vi "Main.vi"(11 "Module Admin":refnum<class "Delacor_lib_QMH_Module Admin.lvclass">) -> ()   [LabVIEW 2018, in "DAQ.lvlib"]
doc: "This template is based off of the Queued Message Handler design pattern and the Queued Message Handler project template that ships with LabVIEW.\n\nThe main difference is that the queue is private to this module and communication between modules is performed via Broadcast and Request events.\n\nRequest events are wrapped in public API methods and are handled in the Event Handling Loop (EHL) of this VI. Any module can register for Broadcast events sent by this module. The EHL generates messages based on user interface actions.\n\nThe Message Handling Loop (MHL) processes messages generated by the EHL, or by other messages. The messages are string values, so new messages can be added easily to the Message Cases case structure in the MHL. Each message cluster can also provide an optional value for Message Data, which is a variant that can be converted to whatever message-specific data is required.\n_____\nBased on DQMH Project Template 6.1.0.94."
uses:
  DAQ.lvlib
  <vilib>/Delacor/Delacor QMH/Libraries/Module Admin_class/Delacor_lib_QMH_Module Admin.lvclass
  Module Data--cluster.ctl
  <vilib>/Modbus/master/Modbus Master.lvclass
  <vilib>/Delacor/Delacor QMH/Libraries/Message Queue_class/Delacor_lib_QMH_Message Queue.lvclass/Delacor_lib_QMH_Message Queue.ctl
  Stop Argument--cluster.ctl
  <vilib>/Delacor/Delacor QMH/Libraries/Module Admin_class/Delacor_lib_QMH_Module Admin.lvclass/Delacor_lib_QMH_Module Admin.ctl
  Update Sampling Rate Argument--cluster.ctl
  <vilib>/Utility/miscctls.llb/LVPointTypeDef.ctl
  <vilib>/Delacor/Delacor QMH/Libraries/Message Queue_class/Delacor_lib_QMH_Enqueue Message (Single).vi
  <vilib>/Delacor/Delacor QMH/Libraries/Module Admin_class/Delacor_lib_QMH_Get External Launch.vi
  <vilib>/Delacor/Delacor QMH/Libraries/Message Queue_class/Delacor_lib_QMH_Enqueue Message (Array).vi
  <vilib>/Utility/error.llb/Error Cluster From Error Code.vi
  <vilib>/ErrorRing/Error Ring.xnode
  <vilib>/Delacor/Delacor QMH/Libraries/Message Queue_class/Delacor_lib_QMH_Message Queue.lvclass
panel:
  out "Message":string
  out "error out":errorcluster
  out "Status":string
  in  "Simulate MHL Error":bool
  in  "Simulate EHL Error":bool
  # "Other QMH Modules communicate with this Module via its Public API (wrappers for its Request Events).\n\nThis Module communicates with other Modules via its Broadcast Events.\nAny module that wants to get these messages, just registers for this module's Broadcast events."
  # "This template is for the Delacor Modified Queued Message Handler design pattern.\n\nSee the block diagram for more information on how to use this template."
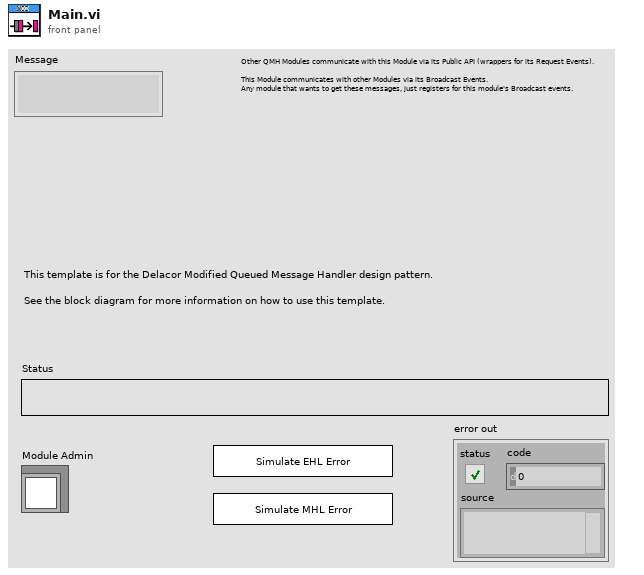
[diagram p1: front panel]
types:
  T1 = typedef "DAQ.lvlib/Request Events--cluster.ctl" = cluster{"Stop Module":refnum<user-event>, "Show Panel":refnum<user-event>, "Hide Panel":refnum<user-event>, "Get Module Execution Status":refnum<user-event>, "Show Diagram":refnum<user-event>, "Wakeup or Sleep HL":refnum<user-event>, "建立连接":refnum<user-event>, "断开连接":refnum<user-event>, "Update Sampling Rate":refnum<user-event>}
  T2 = typedef "DAQ.lvlib/Module Data--cluster.ctl" = cluster{"Status":string, "Mod":cluster{"Con?":bool, "主设备":refnum<class "Modbus Master.lvclass">}, "Sampling Rate":i32}
  T3 = enum32{"invalid lock state", "Not Locked", "Locked (No Password)", "Password-protected"}
  T4 = typedef "DAQ.lvlib/Stop Argument--cluster.ctl" = cluster{"Origin":string, "Exit via Stop Module Req?":bool, "Wait for Module to stop?":bool}
  T5 = typedef "DAQ.lvlib/建立连接 Argument--cluster.ctl" = cluster{"Mod ID":i32}
  T6 = typedef "DAQ.lvlib/断开连接 Argument--cluster.ctl" = cluster{"Mod ID":i32}
  T7 = typedef "DAQ.lvlib/Update Sampling Rate Argument--cluster.ctl" = cluster{"Sampling Rate":i32}
  T8 = typedef "LVPointTypeDef.ctl" = cluster{"Horizontal":i16, "Vertical":i16}
  T9 = enum32{"Invalid", "Standard", "Closed", "Hidden", "Minimized", "Maximized"}
  T10 = cluster{"Con?":bool, "主设备":refnum<class "Modbus Master.lvclass">}
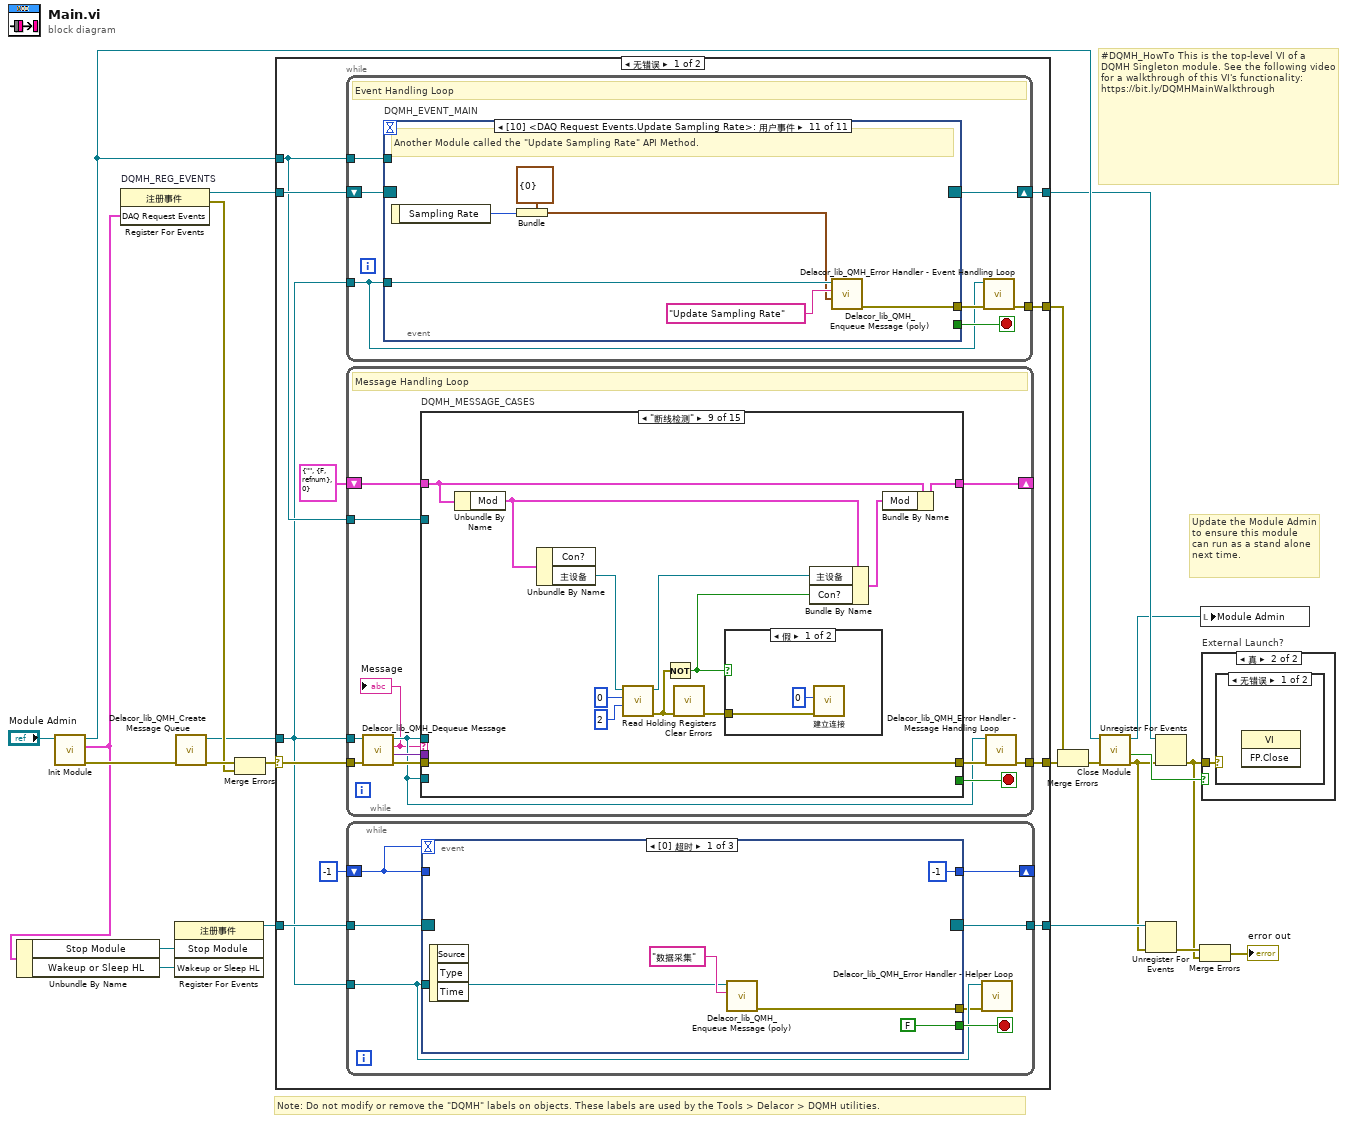
[diagram p0: block diagram]
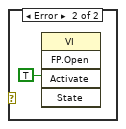
[diagram p3: hidden frame]
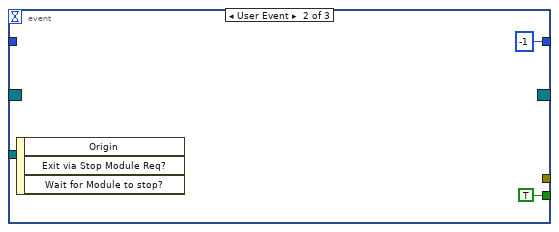
[diagram p4: hidden frame]
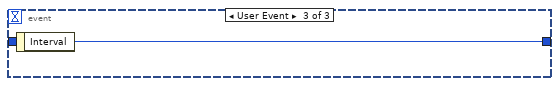
[diagram p5: hidden frame]
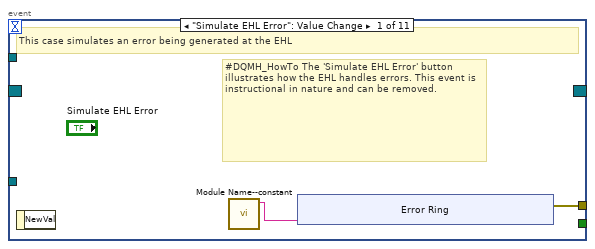
[diagram p6: hidden frame]
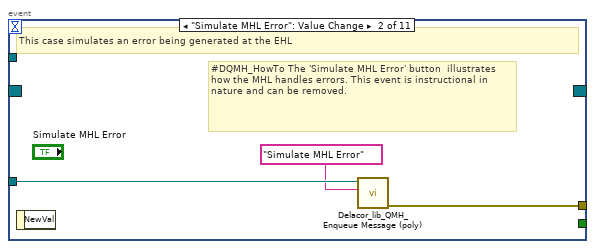
[diagram p7: hidden frame]
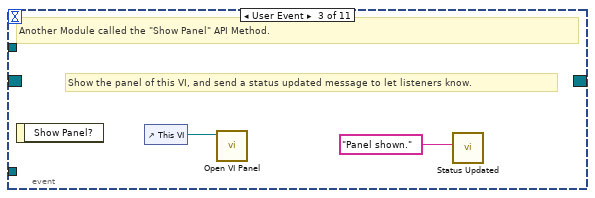
[diagram p8: hidden frame]
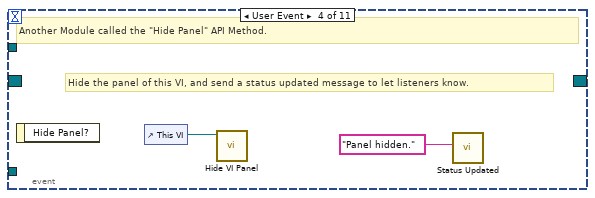
[diagram p9: hidden frame]
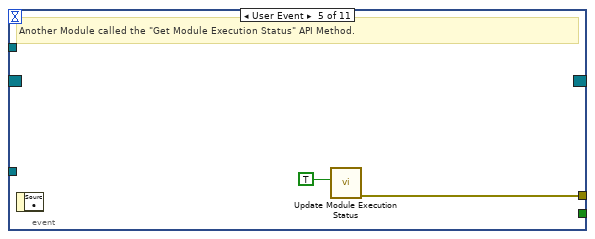
[diagram p10: hidden frame]
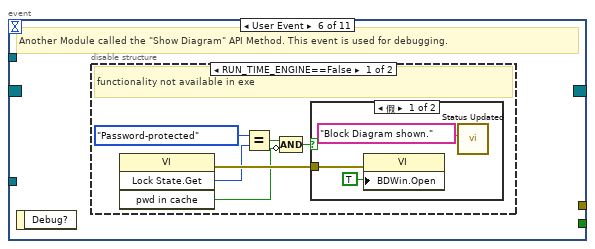
[diagram p11: hidden frame]
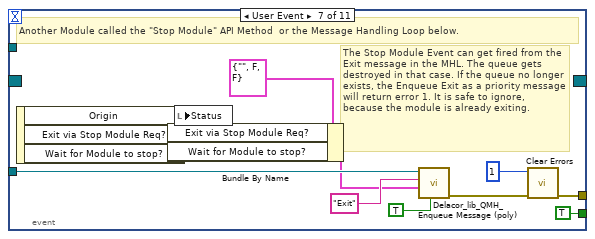
[diagram p14: hidden frame]
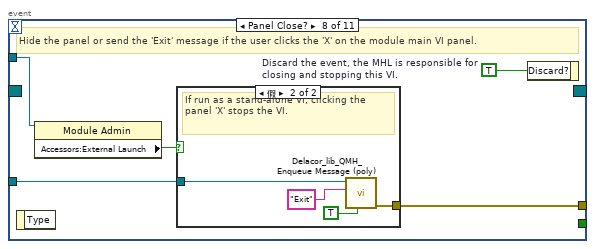
[diagram p15: hidden frame]
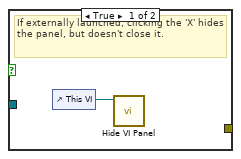
[diagram p16: hidden frame]
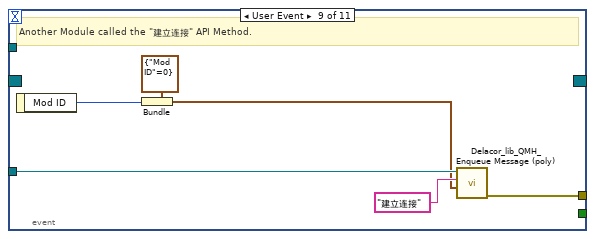
[diagram p17: hidden frame]
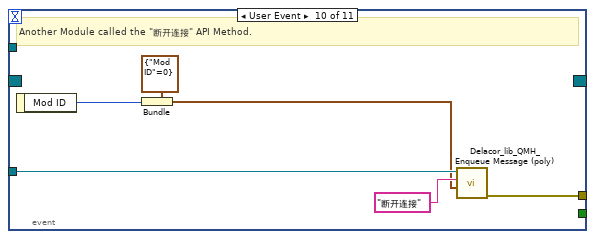
[diagram p18: hidden frame]
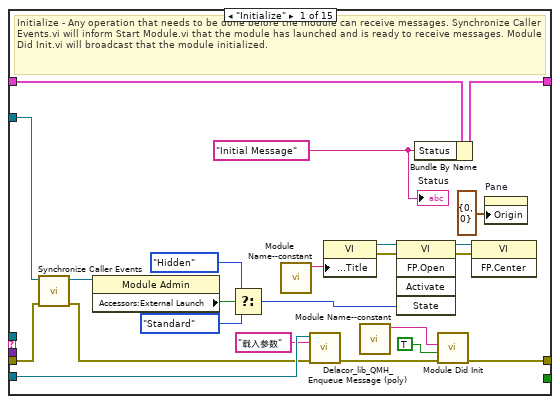
[diagram p19: hidden frame]
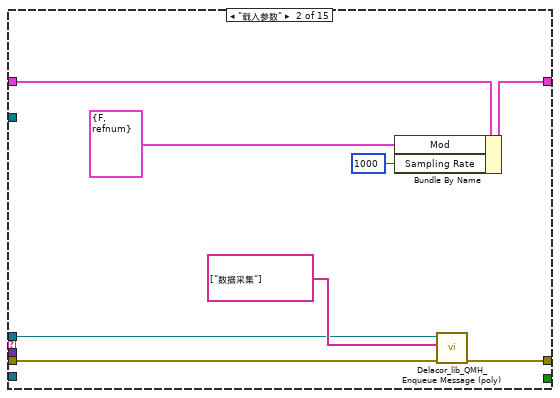
[diagram p20: hidden frame]
diagram:
  # "#DQMH_HowTo This is the top-level VI of a DQMH Singleton module. See the following video for a walkthrough of this VI's functionality: https://bit.ly/DQMHMainWalkthrough"
  # "Note: Do not modify or remove the \"DQMH\" labels on objects. These labels are used by the Tools > Delacor > DQMH utilities."
  # "Update the Module Admin to ensure this module can run as a stand alone next time."
  n1 = call "Init Module.vi"("Singleton Module Admin in"="Module Admin") -> ("error out"=w22:errorcluster, "DAQ Request Events"=w5:T1, "Singleton Module Admin out"=w16:refnum<class "Delacor_lib_QMH_Module Admin.lvclass">)  [unwired: 8 in]
  n2 = Unbundle By Name ("按名称解除捆绑")(w5) -> ("Stop Module"=w8:refnum<user-event>, "Wakeup or Sleep HL"=w7:refnum<user-event>)
  n3 = register-events "DQMH_REG_EVENTS"(w5) -> (reference out=w14:refnum<event-registration>, error out=w17:errorcluster)  [unwired: 2 in]
  n4 = register-events ("注册事件")(w8, w7) -> (reference out=w6:refnum<event-registration>)  [unwired: 2 in, 1 out]
  n5 = call <vilib>:"Delacor_lib_QMH_Create Message Queue.vi"("error in"=w22) -> ("error out"=w19:errorcluster, "Message Queue"=w13:refnum<class "Delacor_lib_QMH_Message Queue.lvclass">)  [unwired: 9 in]
  n6 = Merge Errors(w19, w17) -> (w18:errorcluster)
  n7 = case shown="无错误" w18 {
    selector: w18 -> [w32 w296]
    tunnel: [w34 w295] -> w23
    tunnel: [w31 w301] -> w15
    tunnel: w14 -> [w29 w301]
    tunnel: w13 -> [w25 w294]
    tunnel: [w33 _] -> w21
    tunnel: w16 -> [w28 w297]
    tunnel: w6 -> [w26 w293]
    tunnel: [w24 w293] -> w4
    frame No Error {
      n8 = while {
        tunnel: w25 -> [w50]
        shift-right: [w53] -> w31
        shift-left: w29 -> [w54]
        tunnel: [w55] -> w33
        tunnel: w28 -> [w51]
        stop <- w52 stop-if-true
        # "Event Handling Loop"
        n9 = event "DQMH_EVENT_MAIN" shown="[10] <DAQ Request Events.Update Sampling Rate>: 用户事件" {
          selector: w54 -> [_ _ _ _ _ _ _ _ _ _ _]
          dyn-events: [_ _ _ _ _ _ _ _ _ _ _] -> w53
          timeout: _ -> [_ _ _ _ _ _ _ _ _ _ _]
          tunnel: [_ _ _ _ _ _ TRUE ("Discard?") _ _ _ _] -> w52
          tunnel: w50 -> [_ w67 _ _ _ _ w91 w98 w111 w117 w123]
          tunnel: [w58 w68 _ _ w74 _ w94 w100 w106 w112 w118] -> w56
          tunnel: w51 -> [_ _ _ _ _ _ _ w97 _ _ _]
          event "Simulate EHL Error": Value Change {
            # "#DQMH_HowTo The 'Simulate EHL Error' button  illustrates how the EHL handles errors. This event is instructional in nature and can be removed."
            # "This case simulates an error being generated at the EHL"
            n10 = event-data() -> ()  [unwired: 1 in, 1 out]
            n11 = call "Module Name--constant.vi"() -> ("Module Name"=w57:string)  [unwired: 11 in]
            n12 = xnode "Error Ring"("参数 0"=w57) -> ("错误输出"=w58:errorcluster)
          }
          event "Simulate MHL Error": Value Change {
            # "#DQMH_HowTo The 'Simulate MHL Error' button  illustrates how the MHL handles errors. This event is instructional in nature and can be removed."
            # "This case simulates an error being generated at the EHL"
            n13 = event-data() -> ()  [unwired: 1 in, 1 out]
            n14 = call-poly <vilib>:"Delacor_lib_QMH_Enqueue Message (poly).vi"("Message"="Simulate MHL Error", "Message Queue in"=w67) -> ("error out"=w68:errorcluster)  [unwired: 8 in, 1 out]
          }
          event User Event {
            # "Show the panel of this VI, and send a status updated message to let listeners know."
            # "Another Module called the \"Show Panel\" API Method."
            n15 = event-data() -> ()  [unwired: 1 in, 1 out]
            n16 = control-ref of="This VI"() -> (w70:refnum<vi>)
            n17 = call "Open VI Panel.vi"("VI"=w70) -> ()  [unwired: 10 in, 1 out]
            n18 = call "Status Updated.vi"("Status"="Panel shown." ("format string")) -> ()  [unwired: 10 in, 1 out]
          }
          event User Event {
            # "Hide the panel of this VI, and send a status updated message to let listeners know."
            # "Another Module called the \"Hide Panel\" API Method."
            n19 = event-data() -> ()  [unwired: 1 in, 1 out]
            n20 = control-ref of="This VI"() -> (w72:refnum<vi>)
            n21 = call "Hide VI Panel.vi"("VI"=w72) -> ()  [unwired: 10 in, 1 out]
            n22 = call "Status Updated.vi"("Status"="Panel hidden." ("format string")) -> ()  [unwired: 10 in, 1 out]
          }
          event User Event {
            # "Another Module called the \"Get Module Execution Status\" API Method."
            n23 = event-data() -> ()  [unwired: 1 in, 1 out]
            n24 = call "Update Module Execution Status.vi"("Running?"=TRUE) -> ("error out"=w74:errorcluster)  [unwired: 10 in]
          }
          event User Event {
            # "Another Module called the \"Show Diagram\" API Method. This event is used for debugging."
            n25 = event-data() -> ()  [unwired: 1 in, 1 out]
            n26 = disable-structure shown="RUN_TIME_ENGINE==False" {
              frame condition #0 (active) {
                # "functionality not available in exe"
                n27 = invoke class="VI" method="Lock State.Get"() -> (error out=w80:errorcluster, "Get Lock State"=w79:T3, "pwd in cache"=w76:bool)  [unwired: 4 in, 1 out]
                n28 = Equal?(x=T3."Password-protected", y=w79) -> (x = y?=w77:bool)
                n29 = Compound Arithmetic op=AND(w77, invert w76) -> (w75:bool)
                n30 = case "条件结构" shown="假" w75 {
                  tunnel: w80 -> [w83 _]
                  frame False {
                    n31 = property class="VI"(error in=w83, "BDWin.Open"=TRUE ("Block Diagram Window:Open")) -> ()  [unwired: 1 in, 2 out]
                    n32 = call "Status Updated.vi"("Status"="Block Diagram shown." ("format string")) -> ()  [unwired: 10 in, 1 out]
                  }
                  frame True {
                    # "Password-protected VI, and the password is not in the cache. Do not show the diagram."
                  }
                }
              }
              frame condition #1 {
              }
            }
          }
          event User Event {
            # "The Stop Module Event can get fired from the Exit message in the MHL. The queue gets destroyed in that case. If the queue no longer exists, the Enqueue Exit as a priority message will return error 1. It is safe to ignore, because the module is already exiting."
            # "Another Module called the \"Stop Module\" API Method  or the Message Handling Loop below."
            n33 = event-data() -> ("Origin"=w90:string, "Exit via Stop Module Req?"=w86:bool, "Wait for Module to stop?"=w85:bool)  [unwired: 1 in]
            n34 = Bundle By Name(cluster=T4 {"Origin"="", "Exit via Stop Module Req?"=FALSE, "Wait for Module to stop?"=FALSE} ("Stop Argument"), "Exit via Stop Module Req?"=w86, "Wait for Module to stop?"=w85) -> (w84:T4)
            n35 = local write "Status"(w90) -> ()
            n36 = call-poly <vilib>:"Delacor_lib_QMH_Enqueue Message (poly).vi"("Priority Message? (F)"=TRUE, "Message Data"=w84, "Message"="Exit", "Message Queue in"=w91) -> ("error out"=w95:errorcluster)  [unwired: 6 in, 1 out]
            n37 = call <vilib>:"Clear Errors.vi"("error in (no error)"=w95, "specific error code to clear (0: all)"=1) -> ("error out"=w94:errorcluster)  [unwired: 4 in, 1 out]
          }
          event Panel Close? {
            w99 = TRUE  # Discard the event, the MHL is responsible for closing and stopping this VI.
            # "Hide the panel or send the 'Exit' message if the user clicks the 'X' on the module main VI panel."
            n38 = event-data() -> ()  [unwired: 1 in, 1 out]
            n39 = property class="Module Admin"(reference=w97) -> ("Accessors:External Launch"=w96:bool)  [unwired: 1 in, 2 out]
            n40 = case "条件结构" shown="假" w96 {
              tunnel: w98 -> [_ w104]
              tunnel: [_ w105] -> w100
              frame True {
                # "If externally launched, clicking the 'X' hides the panel, but doesn't close it."
                n41 = control-ref of="This VI"() -> (w101:refnum<vi>)
                n42 = call "Hide VI Panel.vi"("VI"=w101) -> ()  [unwired: 10 in, 1 out]
              }
              frame False {
                # "If run as a stand-alone VI, clicking the panel 'X' stops the VI."
                n43 = call-poly <vilib>:"Delacor_lib_QMH_Enqueue Message (poly).vi"("Priority Message? (F)"=TRUE, "Message"="Exit", "Message Queue in"=w104) -> ("error out"=w105:errorcluster)  [unwired: 7 in, 1 out]
              }
            }
            n44 = event-data("Discard?"=w99) -> ()  [unwired: 1 in, 1 out]
          }
          event User Event {
            # "Another Module called the \"建立连接\" API Method."
            n45 = event-data() -> ("Mod ID"=w107:i32)  [unwired: 1 in]
            n46 = Bundle(cluster=T5 {"Mod ID"=0} ("建立连接 Argument"), "Mod ID"=w107) -> (w108:T5)
            n47 = call-poly <vilib>:"Delacor_lib_QMH_Enqueue Message (poly).vi"("Message Data"=w108, "Message"="建立连接", "Message Queue in"=w111) -> ("error out"=w106:errorcluster)  [unwired: 7 in, 1 out]
          }
          event User Event {
            # "Another Module called the \"断开连接\" API Method."
            n48 = event-data() -> ("Mod ID"=w113:i32)  [unwired: 1 in]
            n49 = Bundle(cluster=T6 {"Mod ID"=0} ("断开连接 Argument"), "Mod ID"=w113) -> (w114:T6)
            n50 = call-poly <vilib>:"Delacor_lib_QMH_Enqueue Message (poly).vi"("Message Data"=w114, "Message"="断开连接", "Message Queue in"=w117) -> ("error out"=w112:errorcluster)  [unwired: 7 in, 1 out]
          }
          event User Event {
            # "Another Module called the \"Update Sampling Rate\" API Method."
            n51 = event-data() -> ("Sampling Rate"=w119:i32)  [unwired: 1 in]
            n52 = Bundle(cluster=T7 {"Sampling Rate"=0} ("Update Sampling Rate Argument"), "Sampling Rate"=w119) -> (w120:T7)
            n53 = call-poly <vilib>:"Delacor_lib_QMH_Enqueue Message (poly).vi"("Message Data"=w120, "Message"="Update Sampling Rate", "Message Queue in"=w123) -> ("error out"=w118:errorcluster)  [unwired: 7 in, 1 out]
          }
        }
        n54 = call-dynamic "Delacor_lib_QMH_Error Handler - Event Handling Loop.vi"("error in"=w56, "Message Queue in"=w50) -> ("dup error in"=w55:errorcluster)  [unwired: 8 in, 1 out]
      }
      n55 = while {
        tunnel: w25 -> [w127]
        shift-right: [w130] -> _
        shift-left: T2 {"Status"="", "Mod"={"Con?"=FALSE, "主设备"=refnum}, "Sampling Rate"=0} ("Data Cluster") -> [w131]
        tunnel: w32 -> [w134]
        tunnel: [w132] -> w34
        tunnel: w28 -> [w126]
        stop <- w129 stop-if-true
        # "Message Handling Loop"
        n56 = call-dynamic "Delacor_lib_QMH_Dequeue Message.vi"("error in"=w134, "Message Queue in"=w127) -> ("error out"=w133:errorcluster, "Message Data"=w128:variant, "Message"=w124:string, "Message Queue out"=w125:refnum<class "Delacor_lib_QMH_Message Queue.lvclass">)  [unwired: 6 in]
        "Message" <- w124
        n57 = case "DQMH_MESSAGE_CASES" shown="\"断线检测\"" w124 {
          selector: w124 -> [_ _ _ _ _ _ _ _ _ _ _ _ _ _ w280]
          tunnel: w125 -> [_ w162 _ _ _ _ _ w207 _ _ _ _ w247 w272 _]
          tunnel: w133 -> [w156 w161 w168 w179 w192 w200 w203 w206 w222 w228 w232 w237 w254 w278 w282]
          tunnel: [w155 w160 w168 w171 w191 w198 w202 w208 w222 w227 w232 w236 w250 w275 w283] -> w135
          tunnel: w131 -> [w146 w166 w167 w175 w187 w199 w201 w210 w221 w230 w231 w234 w249 w264 w281]
          tunnel: [w145 w165 w167 w170 w186 w194 w201 w210 w216 w226 w231 w234 w249 w264 w281] -> w130
          tunnel: [_ _ _ _ _ _ _ _ _ _ _ _ _ w271 _] -> w129
          tunnel: w128 -> [_ _ _ w178 w190 w197 _ _ _ _ _ _ w248 w270 _]
          tunnel: w126 -> [w147 _ _ _ _ _ _ _ _ _ _ _ w246 w265 _]
          tunnel: w125 -> [w139 _ _ _ _ _ _ _ _ _ _ _ _ _ _]
          frame "Initialize" {
            w141 = "Initial Message" ("Initial Message")
            # "Initialize - Any operation that needs to be done before the module can receive messages. Synchronize Caller Events.vi will inform Start Module.vi that the module has launched and is ready to receive messages. Module Did Init.vi will broadcast that the module initialized."
            n58 = call "Synchronize Caller Events.vi"("error in (no error)"=w156, "Singleton Module Admin in"=w147) -> ("error out"=w137:errorcluster, "Singleton Module Admin out"=w142:refnum<class "Delacor_lib_QMH_Module Admin.lvclass">)  [unwired: 8 in]
            n59 = property class="Module Admin"(reference=w142) -> ("Accessors:External Launch"=w151:bool)  [unwired: 1 in, 2 out]
            n60 = Select(t=T9."Hidden" ("State"), s=w151, f=T9."Standard" ("State")) -> (s? t:f=w148:T9)
            n61 = call "Module Name--constant.vi"() -> ("Module Name"=w154:string)  [unwired: 11 in]
            n62 = call-poly <vilib>:"Delacor_lib_QMH_Enqueue Message (poly).vi"("error in"=w137, "Message"="载入参数", "Message Queue in"=w139) -> ("error out"=w136:errorcluster)  [unwired: 7 in, 1 out]
            n63 = property class="VI"("Front Panel.Title"=w154) -> (reference out=w153:refnum<vi>, error out=w158:errorcluster)  [unwired: 2 in]
            n64 = call "Module Name--constant.vi"() -> ("Module Name"=w143:string)  [unwired: 11 in]
            n65 = invoke class="VI" method="FP.Open"(reference=w153, error in=w158, "State"=w148) -> (reference out=w152:refnum<vi>, error out=w157:errorcluster)  [unwired: 2 in, 3 out]
            n66 = Bundle By Name(cluster=w146, "Status"=w141) -> (w145:T2)
            n67 = call "Module Did Init.vi"("error in (no error)"=w136, "Initialized?"=TRUE, "Origin"=w143) -> ("error out"=w155:errorcluster)  [unwired: 8 in]
            n68 = invoke class="VI" method="FP.Center"(reference=w152, error in=w157) -> ()  [unwired: 1 in, 3 out]
            n69 = property on="Pane" class="Pane"("Origin"=T8 {"Horizontal"=0, "Vertical"=0}) -> ()  [unwired: 2 in, 2 out]
            "Status" <- w141
          }
          frame "载入参数" {
            n70 = Bundle By Name(cluster=w166, "Mod"=T10 {"Con?"=FALSE, "主设备"=refnum}, "Sampling Rate"=1000) -> (w165:T2)
            n71 = call-poly <vilib>:"Delacor_lib_QMH_Enqueue Message (poly).vi"("error in"=w161, "Message Array"=string[] ["数据采集"] ("Message"), "Message Queue in"=w162) -> ("error out"=w160:errorcluster)  [unwired: 7 in, 1 out]
          }
          frame "---Module Specific---" {
            # "Separator -- The following cases handle messages specific to this Module."
          }
          frame "建立连接" {
            n72 = Variant To Data(error in=w179, type=T5 {"Mod ID"=0} ("建立连接 Argument"), Variant=w178) -> (data=w176:T5, error out=w172:errorcluster)
            n73 = Unbundle By Name(w175) -> ("Mod"=w174:T10)
            n74 = Unbundle By Name(w176) -> ("Mod ID"=w173:i32)
            n75 = call "Modbus_建立连接.vi"("error in (no error)"=w172, "Mod ID"=w173, "Mod"=w174) -> ("error out"=w171:errorcluster, "Mod 2"=w169:T10)  [unwired: 7 in]
            n76 = Bundle By Name(cluster=w175, "Mod"=w169) -> (w170:T2)
          }
          frame "断开连接" {
            n77 = Variant To Data(error in=w192, type=T6 {"Mod ID"=0} ("断开连接 Argument"), Variant=w190) -> (data=w188:T6, error out=w191:errorcluster)
            n78 = Unbundle By Name(w187) -> ("Mod"=w184:T10)
            n79 = Unbundle By Name(w188) -> ()  [unwired: 1 out]
            n80 = Unbundle By Name(w184) -> ("主设备"=w185:refnum<class "Modbus Master.lvclass">)
            n81 = call-dynamic "Close.vi"("Modbus master in"=w185) -> ("error out"=w180:errorcluster)  [unwired: 10 in]
            n82 = call <vilib>:"Clear Errors.vi"("error in (no error)"=w180) -> ()  [unwired: 5 in, 2 out]
            n83 = Bundle By Name(cluster=w184, "Con?"=FALSE, "主设备"=refnum<class "Modbus Master.lvclass"> refnum ("Modbus master in")) -> (w183:T10)
            n84 = Bundle By Name(cluster=w187, "Mod"=w183) -> (w186:T2)
          }
          frame "Update Sampling Rate" {
            n85 = Variant To Data(error in=w200, type=T7 {"Sampling Rate"=0} ("Update Sampling Rate Argument"), Variant=w197) -> (data=w195:T7, error out=w198:errorcluster)
            n86 = Unbundle By Name(w195) -> ("Sampling Rate"=w193:i32)
            n87 = Bundle By Name(cluster=w199, "Sampling Rate"=w193) -> (w194:T2)
          }
          frame "---Copy This Frame---" {
            # "Duplicate this frame when creating new messages.  Change this comment in the duplicated frame to describe this message."
            n88 = Merge Errors(w203) -> (w202:errorcluster)
          }
          frame "数据采集" {
            n89 = Unbundle By Name(w210) -> ("Sampling Rate"=w209:i32)
            n90 = call-poly <vilib>:"Delacor_lib_QMH_Enqueue Message (poly).vi"("error in"=w206, "Message Array"=string[] ["断线检测", "温度数据采集"] ("Message"), "Message Queue in"=w207) -> ("error out"=w205:errorcluster)  [unwired: 7 in, 1 out]
            n91 = call "Wakeup or Sleep HL.vi"("error in"=w205, "Interval"=w209) -> ("error out"=w208:errorcluster)  [unwired: 9 in]
          }
          frame "断线检测" {
            n92 = Unbundle By Name(w221) -> ("Mod"=w215:T10)
            n93 = Unbundle By Name(w215) -> ("主设备"=w218:refnum<class "Modbus Master.lvclass">)  [unwired: 1 out]
            n94 = call-dynamic "Read Holding Registers.vi"("number of holding registers"=u16 2 ("number of coils"), "starting address"=u16 0, "Modbus master in"=w218) -> ("error out"=w217:errorcluster, "Modbus master out"=w213:refnum<class "Modbus Master.lvclass">)  [unwired: 6 in, 1 out]
            n95 = Not(x=w217) -> (.not. x?=w211:bool)
            n96 = call <vilib>:"Clear Errors.vi"("error in (no error)"=w217) -> ("error out"=w212:errorcluster)  [unwired: 5 in, 1 out]
            n97 = case shown="假" w211 {
              tunnel: w212 -> [w223 _]
              frame False {
                n98 = call "建立连接.vi"("error in"=w223, "Mod ID"=0) -> ()  [unwired: 9 in, 1 out]
              }
              frame True {
              }
            }
            n99 = Bundle By Name(cluster=w215, "主设备"=w213, "Con?"=w211) -> (w214:T10)
            n100 = Bundle By Name(cluster=w221, "Mod"=w214) -> (w216:T2)
          }
          frame "温度数据采集" {
            n101 = Unbundle By Name(w230) -> ("Mod"=w229:T10)
            n102 = call "Modbus_采集温度数据.vi"("error in (no error)"=w228, "Mod"=w229) -> ("error out"=w227:errorcluster, "Mod 2"=w225:T10)  [unwired: 8 in]
            n103 = Bundle By Name(cluster=w230, "Mod"=w225) -> (w226:T2)
          }
          frame "---Exit and Error Handling---" {
            # "Separator - The following cases handle errors and exit messages."
          }
          frame "Simulate MHL Error" {
            # "#DQMH_HowTo The 'Simulate MHL Error' button  illustrates how the MHL handles errors. This event is instructional in nature and can be removed."
            # "Simulate an error occurring at the MHL"
            n104 = call "Module Name--constant.vi"() -> ("Module Name"=w233:string)  [unwired: 11 in]
            n105 = xnode "Error Ring"("参数 0"=w233) -> ("错误输出"=w235:errorcluster)
            n106 = Merge Errors(w237, w235) -> (w236:errorcluster)
          }
          frame "Error" {
            # "#CodeRecommended - If you ever change the name of this \"Error\" message, you'll need to update the name in the Check Loop Error.vi as well."
            # "#CodeRecommended - If the module is running in standalone mode (External Launch = FALSE), this code will pop up an error dialog and call the 'Exit' message if an error occurs. Add more fine-grained error handling here."
            # "Error - Check the error message data and respond accordingly. This message is sent by the \"Error Handler\" VIs at the end of each loop in this application."
            n107 = property class="Module Admin"(reference=w246) -> ("Accessors:External Launch"=w245:bool)  [unwired: 1 in, 2 out]
            n108 = Variant To Data(error in=w254, type=errorcluster {"status"=FALSE, "code"=0, "source"=""} ("error constant"), Variant=w248) -> (data=w255:errorcluster, error out=w252:errorcluster)
            n109 = call "Error Reported.vi"("Error"=w255) -> ()  [unwired: 10 in, 1 out]
            n110 = case shown="假" w245 {
              tunnel: [w260 _] -> w251
              tunnel: w247 -> [w258 _]
              tunnel: w255 -> [w259 _]
              frame False {
                # "If the module is running standalone, then pop up an error dialog and call the \"Exit\" message."
                n111 = call <vilib>:"Simple Error Handler.vi"("error in (no error)"=w259) -> ()  [unwired: 4 in, 5 out]
                n112 = call-poly <vilib>:"Delacor_lib_QMH_Enqueue Message (poly).vi"("Priority Message? (F)"=TRUE, "Message"="Exit", "Message Queue in"=w258) -> ("error out"=w260:errorcluster)  [unwired: 7 in, 1 out]
              }
              frame True {
                # "If the module was launched externally, calling the Error Reported broadcast VI is the only action performed by the \"Error\" message. The module's caller can then process the error appropriately."
              }
            }
            n113 = Merge Errors(w252, w251) -> (w250:errorcluster)
            n114 = local write "error out"(w250) -> ()
          }
          frame "Exit" {
            w269 = 91  # 91: not all Exit messages will have an argument
            w271 = TRUE  # Stop the VI
            # "Release the message queue reference"
            # "Exit - Exit the application."
            n115 = Variant To Data(error in=w278, type=T4 {"Origin"="", "Exit via Stop Module Req?"=FALSE, "Wait for Module to stop?"=FALSE} ("Stop Argument"), Variant=w270) -> (data=w267:T4, error out=w274:errorcluster)
            n116 = call <vilib>:"Clear Errors.vi"("error in (no error)"=w274, "specific error code to clear (0: all)"=w269) -> ("error out"=w277:errorcluster)  [unwired: 4 in, 1 out]
            n117 = Unbundle By Name(w264) -> ("Mod"=w263:T10)
            n118 = Unbundle By Name(w263) -> ("主设备"=w262:refnum<class "Modbus Master.lvclass">)
            n119 = control-ref of="This VI"() -> (w266:refnum<vi>)
            n120 = call-dynamic "Delacor_lib_QMH_Release Message Queue.vi"("error in"=w277, "Message Queue"=w272) -> ("error out"=w276:errorcluster)  [unwired: 9 in]
            n121 = call "Handle Exit.vi"("Stop Argument"=w267, "Admin in"=w265, "VI reference"=w266) -> ("error out"=w273:errorcluster)  [unwired: 7 in, 1 out]
            n122 = Merge Errors(w276, w273) -> (w275:errorcluster)
            n123 = call-dynamic "Close.vi"("Modbus master in"=w262) -> ("error out"=w261:errorcluster)  [unwired: 10 in]
            n124 = call <vilib>:"Clear Errors.vi"("error in (no error)"=w261) -> ()  [unwired: 5 in, 2 out]
          }
          frame Default {
            # "'Default' case only runs if there is a message that isn't defined in any of the other cases.  Output a programming error."
            n125 = call "Module Name--constant.vi"() -> ("Module Name"=w279:string)  [unwired: 11 in]
            n126 = xnode "Error Ring"("参数 0"=w280, "参数 1"=w279) -> ("错误输出"=w284:errorcluster)
            n127 = Merge Errors(w282, w284) -> (w283:errorcluster)
          }
        }
        n128 = call-dynamic "Delacor_lib_QMH_Error Handler - Message Handling Loop.vi"("error in"=w135, "Message Queue in"=w125) -> ("dup error in"=w132:errorcluster)  [unwired: 8 in, 1 out]
      }
      n129 = while {
        shift-right: [w40] -> _
        shift-left: -1 ("Interval") -> [w41]
        tunnel: w26 -> [w38]
        tunnel: [w37] -> w24
        tunnel: w25 -> [w36]
        stop <- w39 stop-if-true
        n130 = event "事件结构" shown="[0] 超时" {
          selector: w38 -> [_ _ _]
          dyn-events: [_ _ _] -> w37
          timeout: w41 -> [_ _ _]
          tunnel: w41 -> [_ _ _]
          tunnel: [-1 ("Interval") -1 w49] -> w40
          tunnel: [FALSE TRUE _] -> w39
          tunnel: w36 -> [w44 _ _]
          tunnel: [w43 _ _] -> w35
          event Timeout {
            n131 = event-data() -> ()  [unwired: 1 in, 3 out]
            n132 = call-poly <vilib>:"Delacor_lib_QMH_Enqueue Message (poly).vi"("Message"="数据采集", "Message Queue in"=w44) -> ("error out"=w43:errorcluster)  [unwired: 8 in, 1 out]
          }
          event User Event {
            n133 = event-data() -> ()  [unwired: 1 in, 3 out]
          }
          event User Event {
            n134 = event-data() -> ("Interval"=w49:i32)  [unwired: 1 in]
          }
        }
        n135 = call-dynamic "Delacor_lib_QMH_Error Handler - Helper Loop.vi"("error in"=w35, "Message Queue in"=w36) -> ()  [unwired: 8 in, 2 out]
      }
    }
    frame Error {
      # "Synchronize Caller Events.vi will inform Start Module.vi that the module has launched and will let the code calling Start Module.vi register for broadcasts and would permit the caller receive the broadcast that an error occurred at launch time."
      n136 = call-dynamic "Delacor_lib_QMH_Release Message Queue.vi"("error in"=w296, "Message Queue"=w294) -> ("error out"=w295:errorcluster)  [unwired: 9 in]
      n137 = call "Synchronize Caller Events.vi"("Singleton Module Admin in"=w297) -> ("error out"=w302:errorcluster)  [unwired: 9 in, 1 out]
      n138 = call "Module Name--constant.vi"() -> ("Module Name"=w300:string)  [unwired: 11 in]
      n139 = Format Into String(format string="An error occurred during initialization. %s is no longer running.", w300) -> (resulting string=w298:string)  [unwired: 2 in, 1 out]
      n140 = Merge Errors(w295, w302) -> (w303:errorcluster)
      n141 = call "Error Reported.vi"("Additional Information"=w298, "Error"=w303) -> ()  [unwired: 9 in, 1 out]
    }
  }
  n142 = Merge Errors(w21, w23) -> (w20:errorcluster)
  n143 = call "Close Module.vi"("error in (no error)"=w20, "Module Admin in"=w16) -> ("error out"=w3:errorcluster, "External Launch"=w10:bool, "Module Admin out"=w11:refnum<class "Delacor_lib_QMH_Module Admin.lvclass">)  [unwired: 7 in]
  n144 = Unregister For Events(event registration refnum=w4, error in=w3) -> (error out=w9:errorcluster)
  n145 = Unregister For Events(event registration refnum=w15, error in=w3) -> (error out=w2:errorcluster)
  n146 = Merge Errors(w9, w2) -> (→"error out":errorcluster)
  n147 = local write "Module Admin"(w11) -> ()
  n148 = case "External Launch?" shown="真" w10 {
    tunnel: w2 -> [_ w304]
    frame False {
    }
    frame True {
      n149 = case "条件结构" shown="无错误" w304 {
        frame No Error {
          n150 = invoke class="VI" method="FP.Close"() -> ()  [unwired: 3 in, 3 out]
        }
        frame Error {
          n151 = invoke class="VI" method="FP.Open"("Activate"=TRUE ("Activate?")) -> ()  [unwired: 4 in, 5 out]
        }
      }
    }
  }
